vi "Flush(DepthProfiling_3D).vi"(0 "data buffer in":refnum<queue>, 1 "Image in":dbl[][][](array[numeric]), 2 "Z Counter":i32, 5 "Image Params":T2={"File Header"={"Start Position"=[], "StepWidth"=[0.05, 0.05], "Dimension"=[], "SpecLength"=10000}, "mzCali."=[0.0, 1.0, 0.0], "m/z_Array"=[0.0, 1.0, 0.0], "SampleRate"=0.0, "TrigDelay"=0.0, "file refnum"=refnum, "file path"=path "", "PeakOI"=[], "Binning"={"Enable"=FALSE, "BinType"=enum."ByScreen", "BinWidth"=0.5, "Maximum"=0.0, "Minimum"=0.0}} {"SampleRate" items=["50MS/s"=50000000.0, "100MS/s"=100000000.0, "125MS/s"=125000000.0, "200MS/s"=200000000.0, "250MS/s"=250000000.0, "500MS/s"=500000000.0, "1GS/s"=1000000000.0, "1.6GS/s"=1600000000.0]}, 7 "DepthProfileBuffer in":T1(array[cluster]), 9 "Y_img":i32, 11 "error in":errorcluster, 12 "conv. coeff.":sgl=655.0) -> (3 "Image out":dbl[][][](array[numeric]), 6 "file refnum out":refnum<file>, 8 "DepthProfileBuffer out":T1(array[cluster]), 15 "error out":errorcluster)   [LabVIEW 2013]
uses:
  ProcessMethods/BioMapConversion/BioMAPWriterCoreParams.ctl
  Files/BinaryHeader.ctl
  ControlDef/SampleRateSelector.ctl
  ProcessMethods/Binning/BinType.ctl
panel:
  out "#element":i32
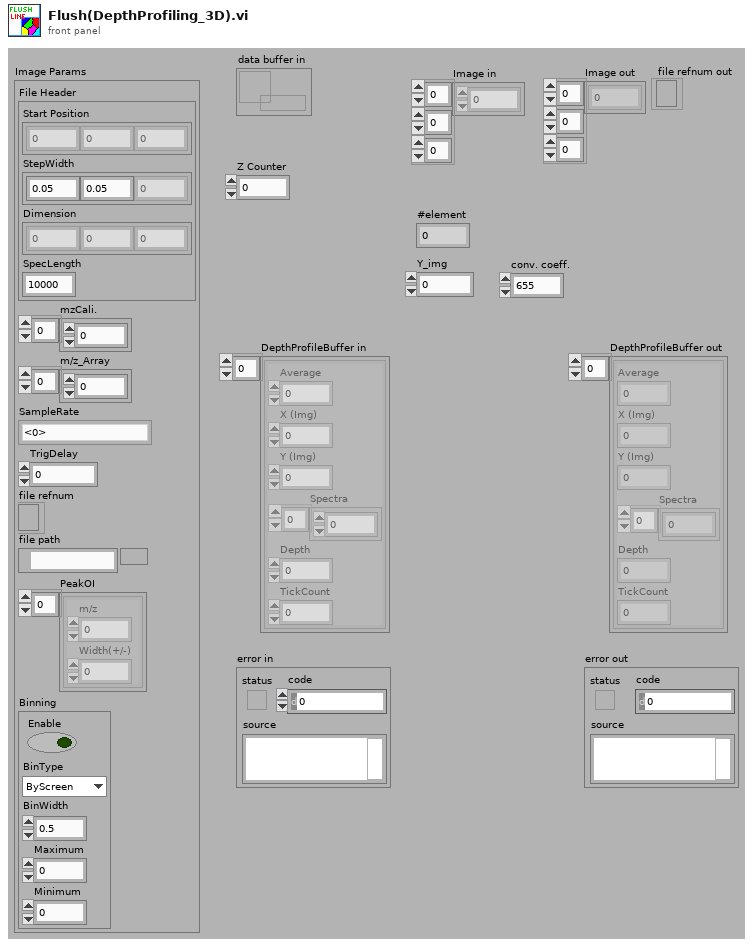
[diagram p1: front panel]
types:
  T1 = cluster{"Average":i32, "X (Img)":i32, "Y (Img)":i32, "Spectra":sgl[], "Depth":i32, "TickCount":dbl}[]
  T2 = typedef "BioMAPWriterCoreParams.ctl" = cluster{"File Header":T3, "mzCali.":dbl[], "m/z_Array":dbl[], "SampleRate":T4, "TrigDelay":dbl, "file refnum":refnum<file>, "file path":path, "PeakOI":cluster{"m/z":dbl, "Width(+/-)":dbl}[], "Binning":cluster{"Enable":bool, "BinType":T5, "BinWidth":dbl, "Maximum":dbl, "Minimum":dbl}}
  T3 = typedef "BinaryHeader.ctl" = cluster{"Start Position":dbl[], "StepWidth":dbl[], "Dimension":i32[], "SpecLength":i32}
  T4 = typedef "SampleRateSelector.ctl" = dbl
  T5 = typedef "BinType.ctl" = enum16{"ByTime", "ByScreen", "ByMass", "ToUnitMass"}
  T6 = enum16{"big-endian, network order", "native, host order", "little-endian"}
  T7 = cluster{"Average":i32, "X (Img)":i32, "Y (Img)":i32, "Spectra":sgl[], "Depth":i32, "TickCount":dbl}
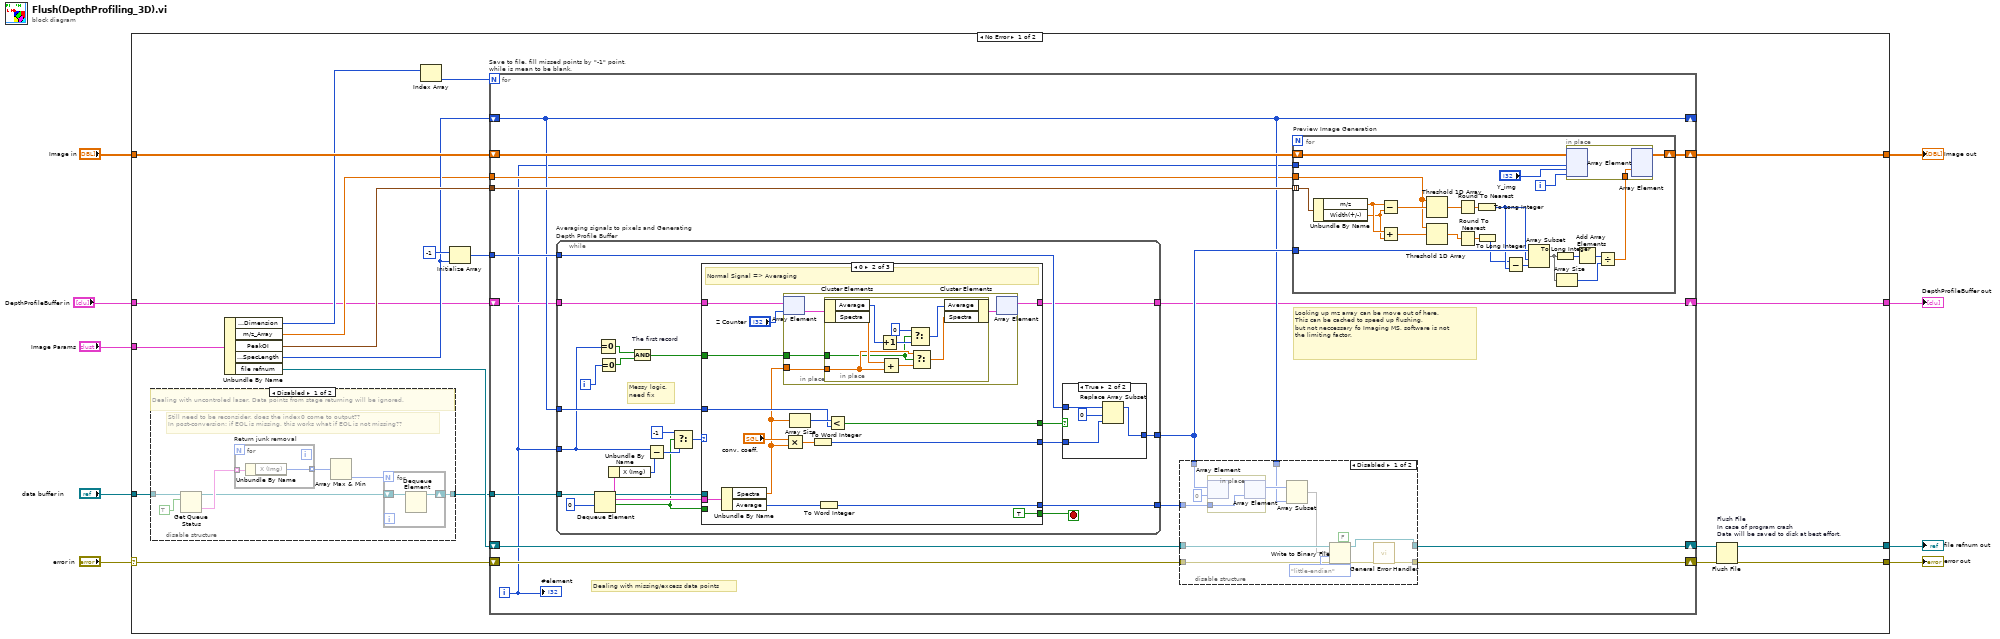
[diagram p0: block diagram]
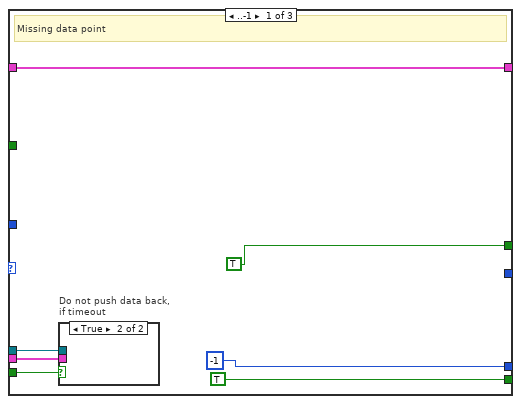
[diagram p5: hidden frame]
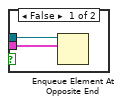
[diagram p6: hidden frame]
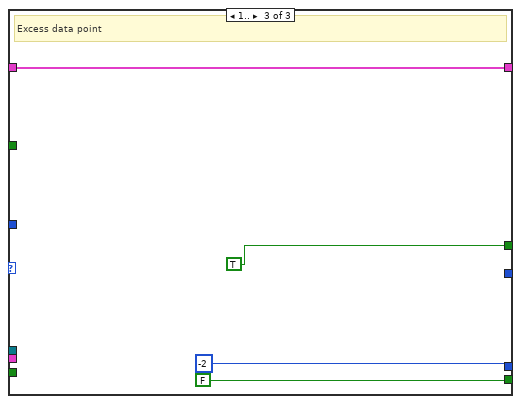
[diagram p7: hidden frame]
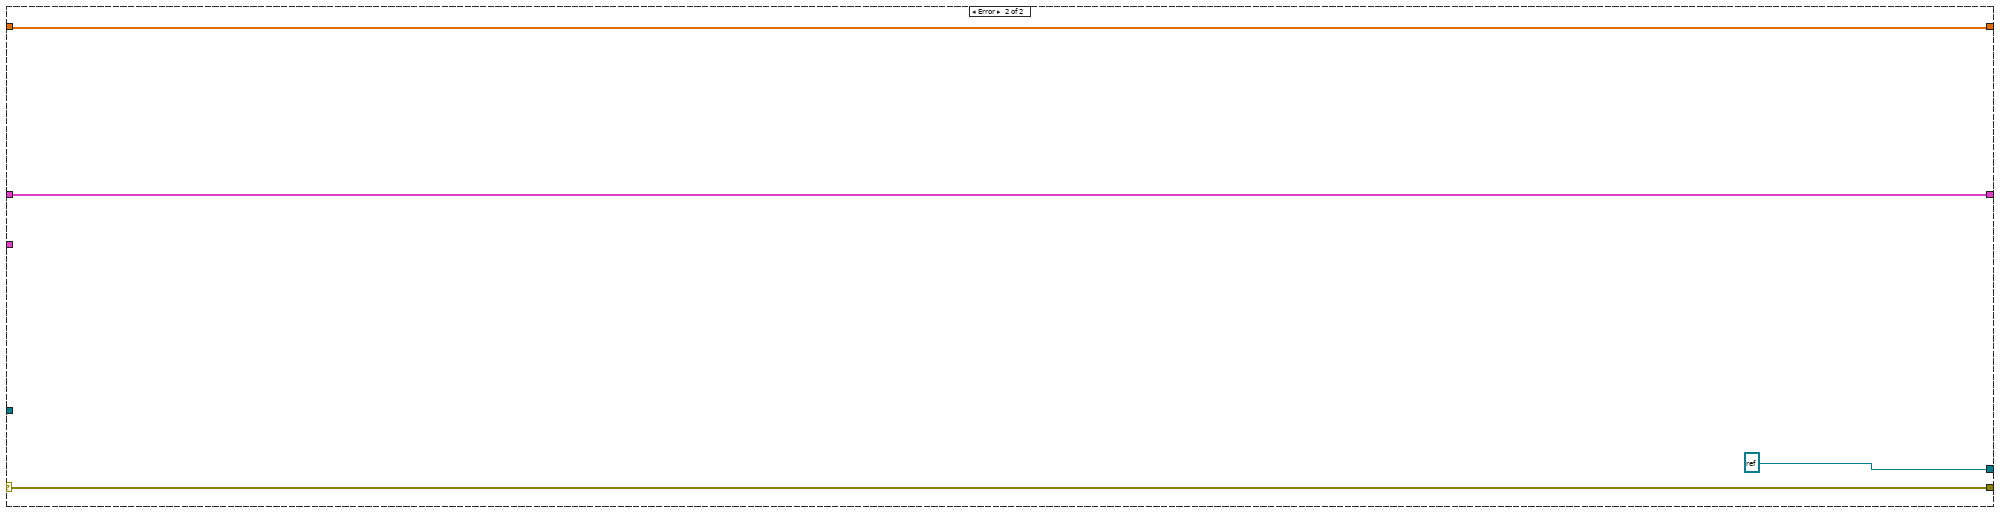
[diagram p8: hidden frame]
diagram:
  n1 = case shown="No Error" "error in" {
    selector: "error in" -> [w26 w171]
    tunnel: [w29 w169] -> w9
    tunnel: [w16 w171] -> w8
    tunnel: [w18 refnum<file> refnum ("file refnum")] -> w7
    tunnel: "Image in" -> [w27 w169]
    tunnel: "data buffer in" -> [w15 _]
    tunnel: "Image Params" -> [w13 _]
    tunnel: "DepthProfileBuffer in" -> [w11 w168]
    tunnel: [w10 w168] -> w1
    frame No Error {
      n2 = disable-structure shown="Disabled" {
        disable-tunnel: w15 -> [w34 w41]
        disable-tunnel: [w32 w41] -> w21
        frame Disabled {
          # "Still need to be reconsider, does the index0 come to output??\nIn post-conversion: if EOL is missing, this works what if EOL is not missing??"
          # "Dealing with uncontroled laser. Data points from stage returning will be ignored."
          n3 = Get Queue Status(queue=w34, return elements? (F)=TRUE) -> (queue out=w33:refnum<queue>, elements=w36:T1)  [unwired: 1 in, 6 out]
          n4 = for "Return junk removal" {
            tunnel: w36 -> [w40] mode=indexing
            tunnel: [w39] -> w31 mode=indexing
            n5 = Unbundle By Name(w40) -> ("X (Img)"=w39:i32)
          }
          n6 = Array Max & Min(array=w31) -> (min index (indices)=w30:i32)  [unwired: 3 out]
          n7 = for {
            N: w30 -> [_]
            shift-right: [w37] -> w32
            shift-left: w33 -> [w38]
            n8 = Dequeue Element(queue=w38) -> (queue out=w37:refnum<queue>)  [unwired: 2 in, 3 out]
          }
        }
        frame Enabled {
          # "batch binning"
        }
      }
      n9 = Unbundle By Name(w13) -> ("File Header.Dimension"=w25:i32[], "m/z_Array"=w12:dbl[], "PeakOI"=w23:cluster{"m/z":dbl, "Width(+/-)":dbl}[], "File Header.SpecLength"=w14:i32, "file refnum"=w24:refnum<file>)
      n10 = Index Array(array=w25) -> (element=w22:i32)  [unwired: 1 in]
      n11 = Initialize Array(i16 -1 ("element"), w14) -> (w19:i16[])
      n12 = for "Save to file, fill missed points by \"-1\" point, while is mean to be blank." {
        N: w22 -> [_]
        shift-right: [w51] -> w17
        shift-left: w26 -> [w47]
        shift-right: [w54] -> w29
        shift-left: w27 -> [w53]
        tunnel: w21 -> [w57]
        shift-right: [w55] -> w28
        shift-left: w24 -> [w56]
        tunnel: w23 -> [w52]
        tunnel: w12 -> [w45]
        tunnel: w19 -> [w48]
        shift-right: [w46] -> _
        shift-left: w14 -> [w46]
        shift-right: [w42] -> w10
        shift-left: w11 -> [w44]
        i -> [w43]
        # "Looking up mz array can be move out of here.\nThis can be cached to speed up flushing, \nbut not neccessary fo Imaging MS, software is not \nthe limiting factor."
        # "Dealing with missing/excess data points"
        n13 = while "Averaging signals to pixels and Generating Depth Profile Buffer" {
          tunnel: w57 -> [w96]
          tunnel: [w90] -> w50
          tunnel: w46 -> [w89]
          tunnel: [w85] -> w49
          tunnel: w43 -> [w78]
          tunnel: w48 -> [w83]
          tunnel: w44 -> [w80]
          tunnel: [w79] -> w42
          i -> [w77]
          stop <- w88 stop-if-true
          # "Messy logic,\nneed fix"
          n14 = Dequeue Element(queue=w96, timeout in ms (-1)=0) -> (queue out=w92:refnum<queue>, element=w91:T7, timed out?=w82:bool)  [unwired: 1 in, 1 out]
          n15 = Equal To 0?(x=w78) -> (x = 0?=w76:bool)
          n16 = Equal To 0?(x=w77) -> (x = 0?=w75:bool)
          n17 = Unbundle By Name(w91) -> ("X (Img)"=w94:i32)
          n18 = And "The first record"(x=w76, y=w75) -> (x .and. y?=w74:bool)
          n19 = Subtract(x=w78, y=w94) -> (x-y=w93:i32)
          n20 = Select(t=-1, s=w82, f=w93) -> (s? t:f=w87:i32)
          n21 = case shown="0" w87 {
            tunnel: w92 -> [w105 _ _]
            tunnel: w91 -> [w104 w125 _]
            tunnel: [i16 -1 ("Average") w123 i16 -2 ("Average")] -> w90
            tunnel: w89 -> [_ w118 _]
            tunnel: [TRUE TRUE FALSE] -> w88
            tunnel: [_ w117 _] -> w84
            tunnel: [TRUE w116 TRUE] -> w81
            tunnel: w82 -> [w103 _ _]
            tunnel: w80 -> [w102 w115 w139]
            tunnel: [w102 w113 w139] -> w79
            tunnel: w74 -> [_ w112 _]
            frame ..-1 {
              # "Missing data point"
              n22 = case "Do not push data back, \nif timeout" shown="True" w103 {
                tunnel: w105 -> [w110 _]
                tunnel: w104 -> [w109 _]
                frame False {
                  n23 = Enqueue Element At Opposite End(queue=w110, element=w109) -> ()  [unwired: 2 in, 3 out]
                }
                frame True {
                }
              }
            }
            frame 0 {
              # "Normal Signal => Averaging"
              n24 = Unbundle By Name(w125) -> ("Spectra"=w114:sgl[], "Average"=w122:i32)
              n25 = in-place {
                in-place-border: w114 -> [w127]
                in-place-border: w112 -> [w126]
                n26 = in-place-array #1(w115, "Z Counter") -> (w129:T7)
                n27 = in-place {
                  in-place-border: w127 -> [w131]
                  in-place-border: w126 -> [w130]
                  n28 = in-place-cluster #2(w129) -> ("Average"=w138:i32, "Spectra"=w133:sgl[])
                  n29 = Increment(x=w138) -> (x+1=w136:i32)
                  n30 = Add(x=w133, y=w131) -> (x+y=w132:sgl[])
                  n31 = Select(t=0, s=w130, f=w136) -> (s? t:f=w137:i32)
                  n32 = Select(t=w131, s=w130, f=w132) -> (s? t:f=w134:sgl[])
                  n33 = in-place-cluster #2("Average"=w137, "Spectra"=w134) -> (w128:T7)
                }
                n34 = in-place-array #1(w128) -> (w113:T1)  [unwired: 1 out]
              }
              n35 = Multiply(x="conv. coeff.", y=w114) -> (x*y=w124:sgl[])
              n36 = Array Size(array=w114) -> (size(s)=w119:i32)
              n37 = To Word Integer(number=w124) -> (16bit integer=w117:i16[])
              n38 = To Word Integer(number=w122) -> (16bit integer=w123:i16)
              n39 = Less?(x=w119, y=w118) -> (x < y?=w116:bool)
            }
            frame 1.. {
              # "Excess data point"
            }
          }
          n40 = case shown="True" w81 {
            tunnel: [w97 w101] -> w85
            tunnel: w84 -> [w97 w99]
            tunnel: w83 -> [_ w100]
            frame False {
            }
            frame True {
              n41 = Replace Array Subset(array=w100, new element=w99, index=0) -> (w101:i16[])
            }
          }
        }
        n42 = disable-structure shown="Disabled" {
          disable-tunnel: w56 -> [w70 w73]
          disable-tunnel: [w69 w73] -> w55
          disable-tunnel: [w68 w72] -> w51
          disable-tunnel: w50 -> [w61 _]
          disable-tunnel: w49 -> [w60 _]
          disable-tunnel: w47 -> [w59 w72]
          disable-tunnel: w46 -> [w58 _]
          frame Disabled {
            n43 = in-place {
              in-place-border: w61 -> [w71]
              n44 = in-place-array #3(w60, 0) -> ()  [unwired: 1 out]
              n45 = in-place-array #3(w71) -> (w62:i16[])  [unwired: 1 out]
            }
            n46 = Array Subset(array=w62, length=w58) -> (w63:i16[])  [unwired: 1 in]
            n47 = Write to Binary File(file (use dialog)=w70, data=w63, error in=w59, 5:FALSE ("prepend array or string size? (T)"), 9:T6."little-endian" ("byte order (0:big-endian, network order)")) -> (refnum out=w69:refnum<file>, error out=w64:errorcluster)  [unwired: 1 in, 1 out]
            n48 = call <vilib>:"General Error Handler.vi"("error in (no error)"=w64) -> ("error out"=w68:errorcluster)  [unwired: 10 in, 4 out]
          }
          frame Enabled {
            # "Disable Image writing, \nno need for depth profiling"
          }
        }
        n49 = for "Preview Image Generation" {
          shift-right: [w153] -> w54
          shift-left: w53 -> [w160]
          tunnel: w52 -> [w166] mode=indexing
          tunnel: w49 -> [w159]
          tunnel: w45 -> [w162]
          tunnel: w43 -> [w146]
          i -> [w145]
          n50 = Unbundle By Name(w166) -> ("m/z"=w165:dbl, "Width(+/-)"=w164:dbl)
          n51 = Subtract(x=w165, y=w164) -> (x-y=w163:dbl)
          n52 = Add(x=w165, y=w164) -> (x+y=w161:dbl)
          n53 = Threshold 1D Array(2:w163, 3:w162) -> (0:w158:dbl)  [unwired: 1 in]
          n54 = Threshold 1D Array(2:w161, 3:w162) -> (0:w157:dbl)  [unwired: 1 in]
          n55 = Round To Nearest(number=w158) -> (nearest integer value=w154:dbl)
          n56 = Round To Nearest(number=w157) -> (nearest integer value=w155:dbl)
          n57 = To Long Integer(number=w154) -> (32bit integer=w152:i32)
          n58 = To Long Integer(number=w155) -> (32bit integer=w151:i32)
          n59 = Subtract(x=w151, y=w152) -> (x-y=w156:i32)
          n60 = Array Subset(array=w159, index=w152, length=w156) -> (w148:i16[])
          n61 = To Long Integer(number=w148) -> (32bit integer=w143:i32[])
          n62 = Array Size(array=w148) -> (size(s)=w149:i32)
          n63 = Add Array Elements(numeric array=w143) -> (sum=w150:i32)
          n64 = Divide(x=w150, y=w149) -> (x/y=w147:dbl)
          n65 = in-place {
            in-place-border: w147 -> [w167]
            n66 = in-place-array #4(w160, w146, "Y_img", w145) -> ()  [unwired: 1 out]
            n67 = in-place-array #4(w167) -> (w153:dbl[][][])  [unwired: 3 out]
          }
        }
        "#element" <- w43
      }
      n68 = Flush File "Flush File\nIn case of program crash\nData will be saved to disk at best effort."(refnum=w28, error in=w17) -> (refnum out=w18:refnum<file>, error out=w16:errorcluster)
    }
    frame Error {
    }
  }
  "Image out" <- w9
  "error out" <- w8
  "file refnum out" <- w7
  "DepthProfileBuffer out" <- w1
